vi "Flatten PDU.vi"(8 "error in":errorcluster, 11 "modbus data unit in":refnum<class "Modbus Data Unit.lvclass">) -> (0 "error out":errorcluster, 3 "Full modbus data unit":u8[](array[numeric]))   [LabVIEW 2012, in "Modbus Data Unit.lvclass"]
uses:
  Modbus Data Unit.lvclass
  Modbus Data Unit.lvclass/Modbus Data Unit.ctl
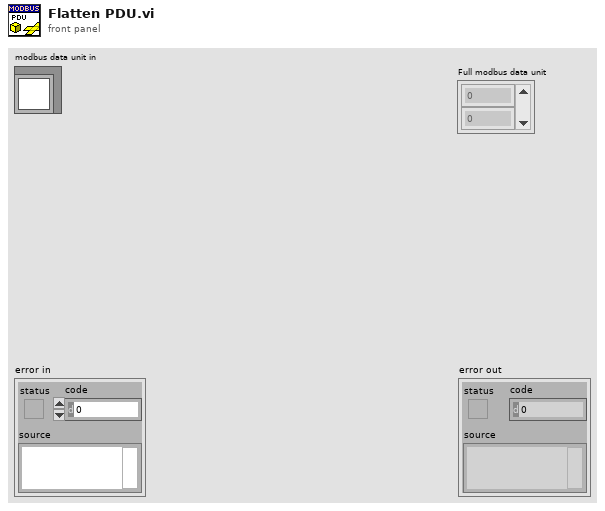
[diagram p1: front panel]
types:
  T1 = typedef "Modbus Data Unit.lvclass/Function.ctl" = u8
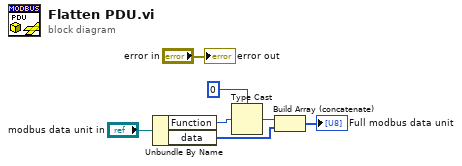
[diagram p0: block diagram]
diagram:
  n1 = Unbundle By Name("modbus data unit in") -> ("Function"=w2:T1, "data"=w1:u8[])
  n2 = Type Cast(type=u8 0, x=w2) -> (*(type *) &x=w4:u8)
  n3 = Build Array (concatenate)(w4, w1) -> (→"Full modbus data unit":u8[])
  "error out" <- "error in"
